vi "室内外单幅图像-阈值设定.vi"() -> ()   [LabVIEW 2018]
uses:
  <vilib>/vision/Image Controls.llb/IMAQ Image.ctl
  <vilib>/Utility/error.llb/DialogType.ctl
  <vilib>/Utility/file.llb/Write Delimited Spreadsheet (I64).vi
  <vilib>/vision/NI_Vision_Development_Module.lvlib
panel:
  out "?":T1(plugin-control)
  in  "刷新按钮":bool
  in  "停止运算":bool
  in  "下一步":bool
  out "Histogram 3":dynamicdata(graph) caption="B直方图"
  out "Histogram 2":dynamicdata(graph) caption="A直方图"
  out "Histogram":dynamicdata(graph) caption="L直方图"
  in  "b颜色通道":cluster{i32, i32}(slide)={-21, 6} scale=-100.0..100.0
  in  "a颜色通道":cluster{i32, i32}(slide)={-21, -7} scale=-100.0..100.0
  in  "L颜色通道":cluster{i32, i32}(slide)={81, 99} scale=0.0..100.0
  out "lie":i32
  out "hang":i32
  out "颜色空间处理后的图，提取火焰":T1(plugin-control)
  in  "Image 4":T1
  out "B":u8[][](array[numeric])
  out "G":u8[][](array[numeric])
  out "R":u8[][](array[numeric])
  out "原图":T1(plugin-control)
  # "Lab颜色空间阈值选择"
  # "Lab颜色分割图像"
  # "滤波平滑图像"
  # "原图"
  # "阈\n值\n选\n择"
  # "火\n焰\n颜\n色\n直\n方\n图"
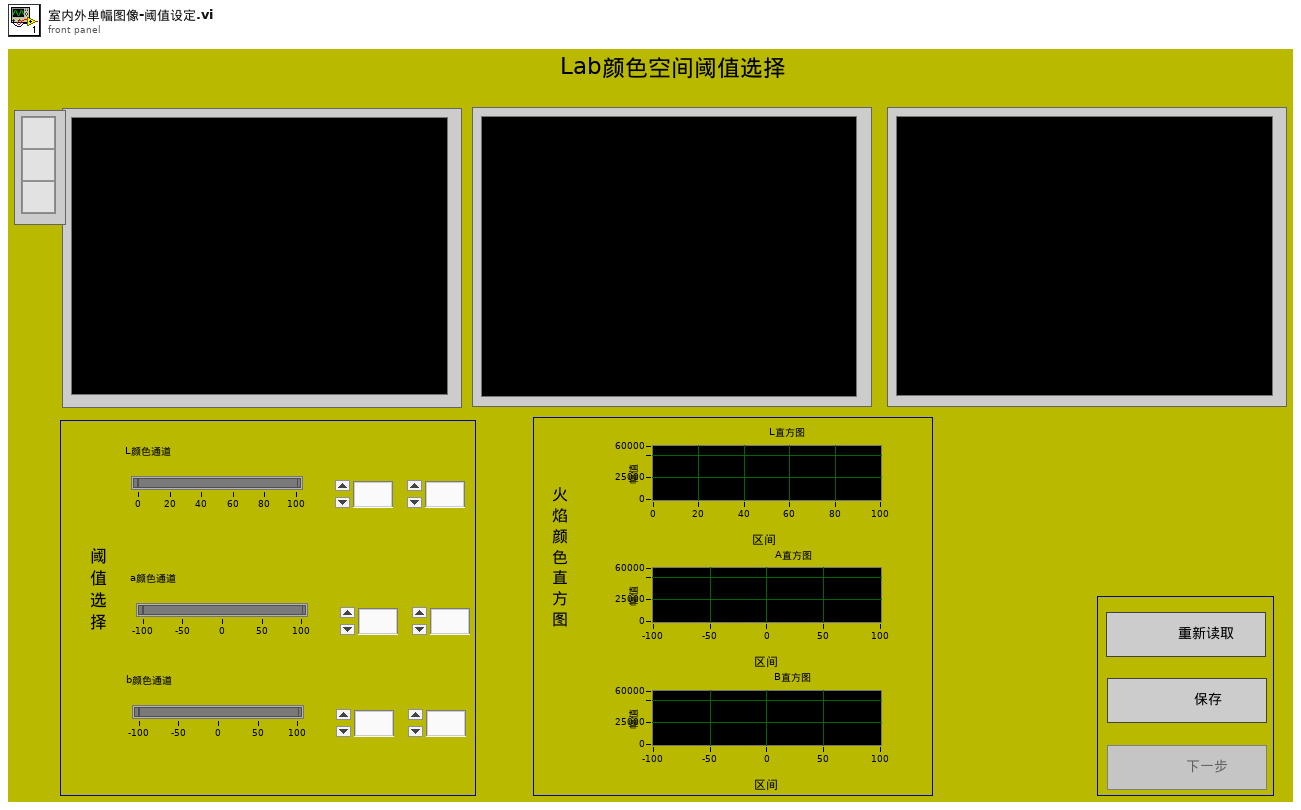
[diagram p1: front panel]
types:
  T1 = typedef "IMAQ Image.ctl" = refnum<image>
  T2 = enum8{"Enabled", "Disabled", "Disabled and Grayed Out"}
  T3 = enum32{"Invalid", "Standard", "Closed", "Hidden", "Minimized", "Maximized"}
  T4 = typedef "Image Type" = u32
  T5 = typedef "DialogType.ctl" = u16
  T6 = cluster{"Global Rectangle":i32[], "Contours":cluster{"Contour Type":u32, "ROI Type":u32, "Points":i32[]}[]}
  T7 = typedef "IMAQ Rectangle" = cluster{"Left":i32, "Top":i32, "Right":i32, "Bottom":i32, "Rotation":dbl}
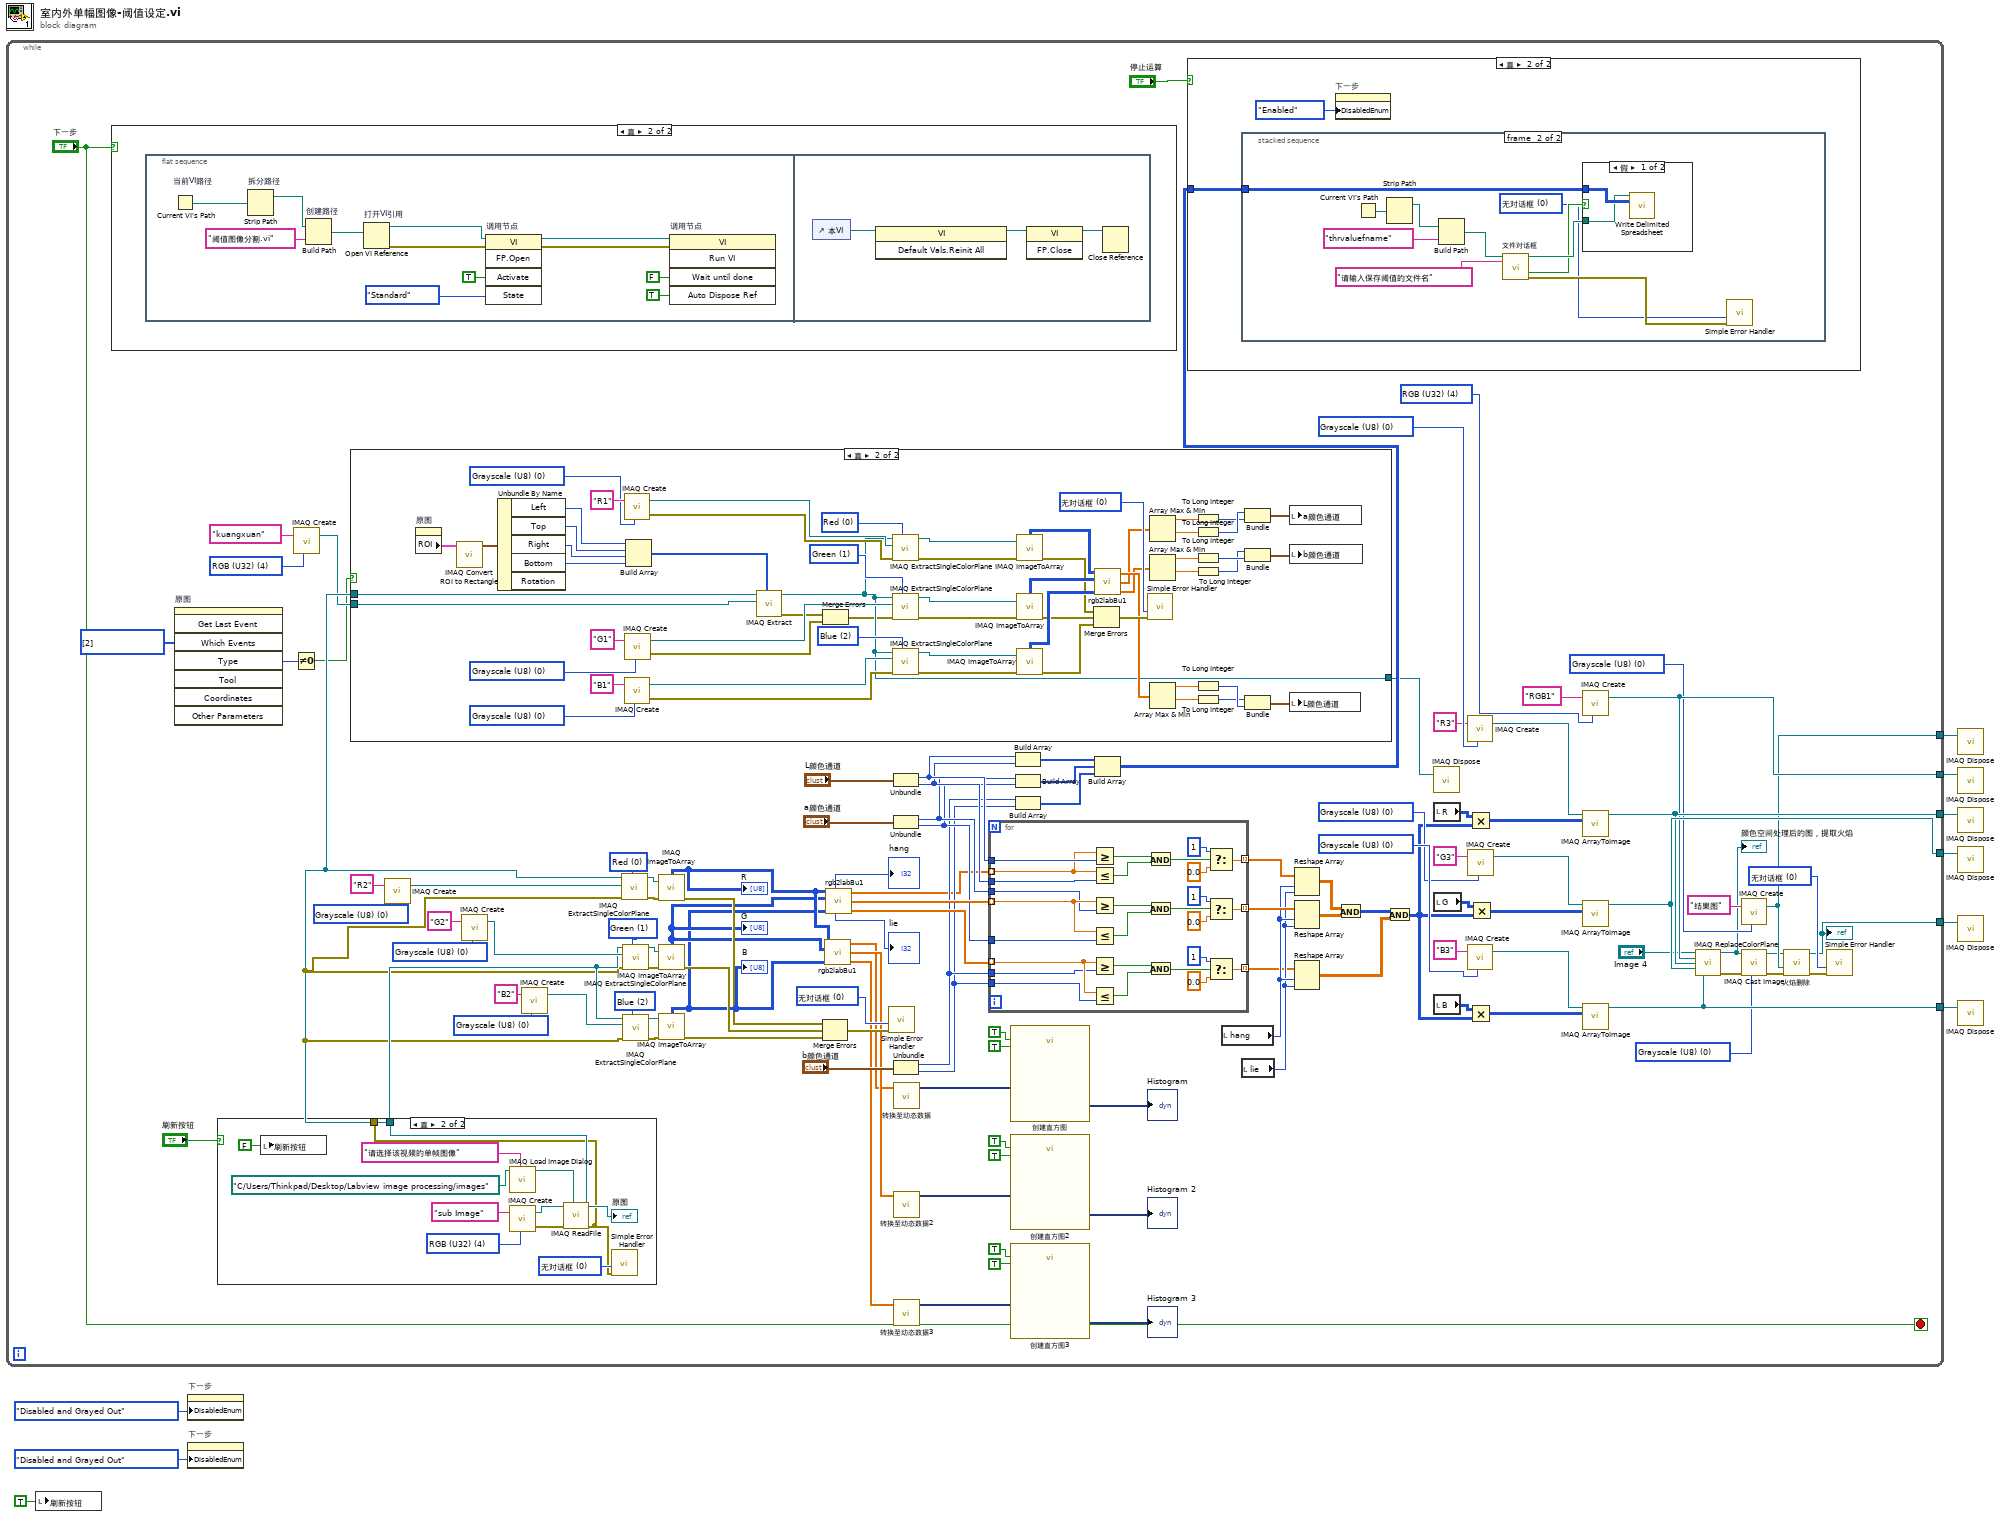
[diagram p0: block diagram]
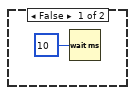
[diagram p2: hidden frame]
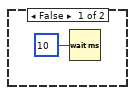
[diagram p3: hidden frame]
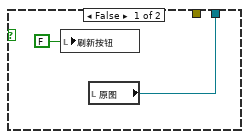
[diagram p4: hidden frame]
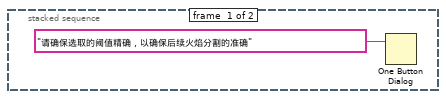
[diagram p6: hidden frame]
diagram:
  n1 = while {
    tunnel: [w123] -> w8
    tunnel: [w122] -> w7
    tunnel: [w121] -> w6
    tunnel: [w120] -> w5
    tunnel: [w119] -> w4
    tunnel: [w11] -> w1
    stop <- "下一步" stop-if-true
    w17 = T4 4 items=["Grayscale (U8)", "Grayscale (I16)", "Grayscale (SGL)", "Complex (CSG)", "RGB (U32)", "HSL (U32)", "RGB (U64)", "Grayscale (U16)"] ("Image Type")
    w16 = i32[] [2] items=["No  event", "Click event", "Draw event", "Move event", "Size event", "Scroll event", "Activate event", "Close event", "Double click event"] ("Events list (all)")
    w28 = T4 0 items=["Grayscale (U8)", "Grayscale (I16)", "Grayscale (SGL)", "Complex (CSG)", "RGB (U32)", "HSL (U32)", "RGB (U64)", "Grayscale (U16)"] ("Image Type")
    w26 = T4 0 items=["Grayscale (U8)", "Grayscale (I16)", "Grayscale (SGL)", "Complex (CSG)", "RGB (U32)", "HSL (U32)", "RGB (U64)", "Grayscale (U16)"] ("Image Type")
    w24 = T4 0 items=["Grayscale (U8)", "Grayscale (I16)", "Grayscale (SGL)", "Complex (CSG)", "RGB (U32)", "HSL (U32)", "RGB (U64)", "Grayscale (U16)"] ("Image Type")
    w54 = T5 0 items=["无对话框", "确定信息", "继续或停止信息", "确定信息＋警告", "继续/停止+警告"] ("type of dialog (OK msg:1)")
    w76 = T4 0 items=["Grayscale (U8)", "Grayscale (I16)", "Grayscale (SGL)", "Complex (CSG)", "RGB (U32)", "HSL (U32)", "RGB (U64)", "Grayscale (U16)"] ("Image Type")
    w77 = T4 4 items=["Grayscale (U8)", "Grayscale (I16)", "Grayscale (SGL)", "Complex (CSG)", "RGB (U32)", "HSL (U32)", "RGB (U64)", "Grayscale (U16)"] ("Image Type")
    w92 = T4 0 items=["Grayscale (U8)", "Grayscale (I16)", "Grayscale (SGL)", "Complex (CSG)", "RGB (U32)", "HSL (U32)", "RGB (U64)", "Grayscale (U16)"] ("Image Type")
    w98 = T4 0 items=["Grayscale (U8)", "Grayscale (I16)", "Grayscale (SGL)", "Complex (CSG)", "RGB (U32)", "HSL (U32)", "RGB (U64)", "Grayscale (U16)"] ("Image Type")
    w96 = T4 0 items=["Grayscale (U8)", "Grayscale (I16)", "Grayscale (SGL)", "Complex (CSG)", "RGB (U32)", "HSL (U32)", "RGB (U64)", "Grayscale (U16)"] ("Image Type")
    w101 = T4 0 items=["Grayscale (U8)", "Grayscale (I16)", "Grayscale (SGL)", "Complex (CSG)", "RGB (U32)", "HSL (U32)", "RGB (U64)", "Grayscale (U16)"] ("Image Type")
    w103 = T5 0 items=["无对话框", "确定信息", "继续或停止信息", "确定信息＋警告", "继续/停止+警告"] ("type of dialog (OK msg:1)")
    w112 = 2 items=["Red", "Green", "Blue", "Hue", "Saturation", "Luminance", "Value", "Intensity"] ("Color Plane")
    w113 = 1 items=["Red", "Green", "Blue", "Hue", "Saturation", "Luminance", "Value", "Intensity"] ("Color Plane")
    w114 = 0 items=["Red", "Green", "Blue", "Hue", "Saturation", "Luminance", "Value", "Intensity"] ("Color Plane")
    n2 = case shown="真" "下一步" {
      frame False {
        n3 = Wait (ms)(milliseconds to wait=u32 10 ("等待时间（毫秒）")) -> ()  [unwired: 1 out]
      }
      frame True {
        n4 = flat-sequence {
          frame #0 {
            n5 = Current VI's Path "当前VI路径"() -> (path=w133:path)
            n6 = Strip Path "拆分路径"(path=w133) -> (stripped path=w136:path)  [unwired: 1 out]
            n7 = Build Path "创建路径"(base path=w136, name or relative path="阈值图像分割.vi" ("名称或相对路径")) -> (appended path=w134:path)
            n8 = Open VI Reference "打开VI引用"(vi path=w134) -> (vi reference=w131:refnum<vi>, error out=w130:errorcluster)  [unwired: 5 in]
            n9 = invoke on="调用节点" class="VI" method="FP.Open"(reference=w131, error in=w130, "Activate"=TRUE ("激活？"), "State"=T3."Standard" ("状态")) -> (reference out=w129:refnum<vi>, error out=w128:errorcluster)  [unwired: 1 in, 3 out]
            n10 = invoke on="调用节点" class="VI" method="Run VI"(reference=w129, error in=w128, "Wait until done"=FALSE ("结束前等待"), "Auto Dispose Ref"=TRUE ("自动销毁引用")) -> ()  [unwired: 1 in, 5 out]
          }
          frame #1 {
            n11 = control-ref of="本VI"() -> (w139:refnum<vi>)
            n12 = invoke class="VI" method="Default Vals.Reinit All"(reference=w139) -> (reference out=w138:refnum<vi>)  [unwired: 2 in, 2 out]
            n13 = invoke class="VI" method="FP.Close"(reference=w138) -> (reference out=w137:refnum<vi>)  [unwired: 2 in, 2 out]
            n14 = Close Reference(reference=w137) -> ()  [unwired: 1 in, 1 out]
          }
        }
      }
    }
    n15 = invoke on="原图" class="ImageControl" method="Get Last Event"("Which Events"=w16) -> ("Type"=w15:i32)  [unwired: 7 in, 7 out]
    n16 = case shown="真" "刷新按钮" {
      tunnel: [_ w203] -> w10
      tunnel: [w201 w204] -> w20
      frame False {
        n17 = local write "刷新按钮"(FALSE ("布尔")) -> ()
        n18 = local read "原图"() -> (w201:T1)
      }
      frame True {
        w208 = T5 0 items=["无对话框", "确定信息", "继续或停止信息", "确定信息＋警告", "继续/停止+警告"] ("type of dialog (OK msg:1)")
        w211 = T4 4 items=["Grayscale (U8)", "Grayscale (I16)", "Grayscale (SGL)", "Complex (CSG)", "RGB (U32)", "HSL (U32)", "RGB (U64)", "Grayscale (U16)"] ("Image Type")
        n19 = local write "刷新按钮"(FALSE ("布尔")) -> ()
        n20 = call "IMAQ Load Image Dialog"("Prompt"="请选择该视频的单帧图像", "Start Path"=path "C:/Users/Thinkpad/Desktop/Labview image processing/images") -> ("Path"=w205:path)  [unwired: 7 in, 2 out]
        n21 = call "IMAQ Create"("Image Name"="sub Image", "Image Type"=w211) -> ("New Image"=w210:T1, "error out"=w209:errorcluster)  [unwired: 2 in, 1 out]
        n22 = call "IMAQ ReadFile"("File Path"=w205, "error in (no error)"=w209, "Image"=w210) -> ("error out"=w203:errorcluster, "Image Out"=w204:T1)  [unwired: 4 in, 3 out]
        "原图" <- w204
        n23 = call <vilib>:"Simple Error Handler.vi"("type of dialog (OK msg:1)"=w208, "error in (no error)"=w203) -> ()  [unwired: 3 in, 5 out]
      }
    }
    n24 = call "IMAQ Create"("Image Name"="kuangxuan", "Image Type"=w17) -> ("New Image"=w19:T1)  [unwired: 2 in, 2 out]
    n25 = Not Equal To 0?(x=w15) -> (x != 0?=w14:bool)
    n26 = case shown="真" w14 {
      tunnel: w19 -> [_ w146]
      tunnel: [_ w145] -> w13
      tunnel: w20 -> [_ w144]
      frame False {
        n27 = Wait (ms)(milliseconds to wait=u32 10) -> ()  [unwired: 1 out]
      }
      frame True {
        w176 = T5 0 items=["无对话框", "确定信息", "继续或停止信息", "确定信息＋警告", "继续/停止+警告"] ("type of dialog (OK msg:1)")
        w187 = 2 items=["Red", "Green", "Blue", "Hue", "Saturation", "Luminance", "Value", "Intensity"] ("Color Plane")
        w188 = 1 items=["Red", "Green", "Blue", "Hue", "Saturation", "Luminance", "Value", "Intensity"] ("Color Plane")
        w189 = 0 items=["Red", "Green", "Blue", "Hue", "Saturation", "Luminance", "Value", "Intensity"] ("Color Plane")
        w193 = T4 0 items=["Grayscale (U8)", "Grayscale (I16)", "Grayscale (SGL)", "Complex (CSG)", "RGB (U32)", "HSL (U32)", "RGB (U64)", "Grayscale (U16)"] ("Image Type")
        w195 = T4 0 items=["Grayscale (U8)", "Grayscale (I16)", "Grayscale (SGL)", "Complex (CSG)", "RGB (U32)", "HSL (U32)", "RGB (U64)", "Grayscale (U16)"] ("Image Type")
        w197 = T4 0 items=["Grayscale (U8)", "Grayscale (I16)", "Grayscale (SGL)", "Complex (CSG)", "RGB (U32)", "HSL (U32)", "RGB (U64)", "Grayscale (U16)"] ("Image Type")
        n28 = property on="原图" class="ImageControl"() -> ("ROI"=w147:T6)  [unwired: 2 in, 2 out]
        n29 = call "IMAQ Convert ROI to Rectangle"("ROI Descriptor"=w147) -> ("Rectangle"=w153:T7)  [unwired: 8 in, 1 out]
        n30 = Unbundle By Name(w153) -> ("Left"=w152:i32, "Top"=w151:i32, "Right"=w150:i32, "Bottom"=w149:i32)  [unwired: 1 out]
        n31 = call "IMAQ Create"("Image Name"="R1", "Image Type"=w197) -> ("New Image"=w192:T1, "error out"=w182:errorcluster)  [unwired: 2 in, 1 out]
        n32 = call "IMAQ Create"("Image Name"="B1", "Image Type"=w193) -> ("New Image"=w190:T1, "error out"=w199:errorcluster)  [unwired: 2 in, 1 out]
        n33 = call "IMAQ Create"("Image Name"="G1", "Image Type"=w195) -> ("New Image"=w191:T1, "error out"=w142:errorcluster)  [unwired: 2 in, 1 out]
        n34 = Build Array(w152, w151, w150, w149) -> (w148:i32[])
        n35 = call "IMAQ Extract"("Optional Rectangle"=w148, "Image Dst"=w146, "Image Src"=w144) -> ("error out"=w143:errorcluster, "Image Dst Out"=w145:T1)  [unwired: 7 in]
        n36 = Merge Errors(w143, w142) -> (w141:errorcluster)
        n37 = call "IMAQ ExtractSingleColorPlane"("Color Plane"=w189, "error in (no error)"=w182, "Image Dst"=w192, "Image Src"=w145) -> ("error out"=w181:errorcluster, "Image Dst Out"=w156:T1)  [unwired: 6 in]
        n38 = call "IMAQ ExtractSingleColorPlane"("Color Plane"=w188, "error in (no error)"=w141, "Image Dst"=w191, "Image Src"=w145) -> ("error out"=w183:errorcluster, "Image Dst Out"=w155:T1)  [unwired: 6 in]
        n39 = call "IMAQ ExtractSingleColorPlane"("Color Plane"=w187, "error in (no error)"=w199, "Image Dst"=w190, "Image Src"=w145) -> ("error out"=w180:errorcluster, "Image Dst Out"=w154:T1)  [unwired: 6 in]
        n40 = call "IMAQ ImageToArray"("error in (no error)"=w181, "Image"=w156) -> ("error out"=w179:errorcluster, "Image Pixels (U8)"=w186:u8[][])  [unwired: 2 in, 3 out]
        n41 = call "IMAQ ImageToArray"("error in (no error)"=w183, "Image"=w155) -> ("error out"=w178:errorcluster, "Image Pixels (U8)"=w185:u8[][])  [unwired: 2 in, 3 out]
        n42 = call "IMAQ ImageToArray"("error in (no error)"=w180, "Image"=w154) -> ("error out"=w177:errorcluster, "Image Pixels (U8)"=w184:u8[][])  [unwired: 2 in, 3 out]
        n43 = Merge Errors(w179, w178, w177) -> (w175:errorcluster)
        n44 = call "rgb2labBu1.vi"("R"=w186, "G"=w185, "B"=w184) -> ("LZ"=w169:dbl[], "aZ"=w158:dbl[], "bZ"=w157:dbl[])  [unwired: 1 in, 2 out]
        n45 = call <vilib>:"Simple Error Handler.vi"("type of dialog (OK msg:1)"=w176, "error in (no error)"=w175) -> ()  [unwired: 3 in, 5 out]
        n46 = Array Max & Min(array=w158) -> (max value=w164:dbl, min value=w165:dbl)  [unwired: 2 out]
        n47 = Array Max & Min(array=w157) -> (max value=w163:dbl, min value=w162:dbl)  [unwired: 2 out]
        n48 = Array Max & Min(array=w169) -> (max value=w174:dbl, min value=w173:dbl)  [unwired: 2 out]
        n49 = To Long Integer(number=w164) -> (32bit integer=w167:i32)
        n50 = To Long Integer(number=w165) -> (32bit integer=w168:i32)
        n51 = To Long Integer(number=w163) -> (32bit integer=w160:i32)
        n52 = To Long Integer(number=w162) -> (32bit integer=w159:i32)
        n53 = To Long Integer(number=w174) -> (32bit integer=w171:i32)
        n54 = To Long Integer(number=w173) -> (32bit integer=w170:i32)
        n55 = Bundle(w168, w167) -> (w166:cluster{i32, i32})  [unwired: 1 in]
        n56 = Bundle(w159, w160) -> (w161:cluster{i32, i32})  [unwired: 1 in]
        n57 = Bundle(w170, w171) -> (w172:cluster{i32, i32})  [unwired: 1 in]
        n58 = local write "a颜色通道"(w166) -> ()
        n59 = local write "b颜色通道"(w161) -> ()
        n60 = local write "L颜色通道"(w172) -> ()
      }
    }
    n61 = call "IMAQ Create"("Image Name"="R2", "Image Type"=w24) -> ("New Image"=w21:T1)  [unwired: 2 in, 2 out]
    n62 = call "IMAQ Create"("Image Name"="G2", "Image Type"=w26) -> ("New Image"=w22:T1)  [unwired: 2 in, 2 out]
    n63 = call "IMAQ Create"("Image Name"="B2", "Image Type"=w28) -> ("New Image"=w23:T1)  [unwired: 2 in, 2 out]
    n64 = call "IMAQ ExtractSingleColorPlane"("Color Plane"=w114, "error in (no error)"=w10, "Image Dst"=w21, "Image Src"=w20) -> ("error out"=w108:errorcluster, "Image Dst Out"=w118:T1)  [unwired: 6 in]
    n65 = call "IMAQ ExtractSingleColorPlane"("Color Plane"=w113, "error in (no error)"=w10, "Image Dst"=w22, "Image Src"=w20) -> ("error out"=w109:errorcluster, "Image Dst Out"=w117:T1)  [unwired: 6 in]
    n66 = call "IMAQ ExtractSingleColorPlane"("Color Plane"=w112, "error in (no error)"=w10, "Image Dst"=w23, "Image Src"=w20) -> ("error out"=w107:errorcluster, "Image Dst Out"=w52:T1)  [unwired: 6 in]
    n67 = call "IMAQ ImageToArray"("error in (no error)"=w108, "Image"=w118) -> ("error out"=w106:errorcluster, "Image Pixels (U8)"=w40:u8[][])  [unwired: 2 in, 3 out]
    "R" <- w40
    n68 = call "IMAQ ImageToArray"("error in (no error)"=w109, "Image"=w117) -> ("error out"=w105:errorcluster, "Image Pixels (U8)"=w39:u8[][])  [unwired: 2 in, 3 out]
    "G" <- w39
    n69 = call "IMAQ ImageToArray"("error in (no error)"=w107, "Image"=w52) -> ("error out"=w104:errorcluster, "Image Pixels (U8)"=w38:u8[][])  [unwired: 2 in, 3 out]
    "B" <- w38
    n70 = Merge Errors(w106, w105, w104) -> (w102:errorcluster)
    n71 = call "rgb2labBu1.vi"("R"=w40, "G"=w39, "B"=w38) -> ("LZ"=w37:dbl[], "aZ"=w42:dbl[], "bZ"=w46:dbl[])  [unwired: 1 in, 2 out]
    n72 = call "rgb2labBu1.vi"("R"=w40, "G"=w39, "B"=w38) -> ("hang"=→"hang":i32, "lie"=→"lie":i32, "LZ"=w51:dbl[], "aZ"=w115:dbl[], "bZ"=w116:dbl[])  [unwired: 1 in]
    n73 = call <vilib>:"Simple Error Handler.vi"("type of dialog (OK msg:1)"=w103, "error in (no error)"=w102) -> ()  [unwired: 3 in, 5 out]
    n74 = Unbundle("L颜色通道") -> (w66:i32, w65:i32)
    n75 = Unbundle("a颜色通道") -> (w64:i32, w63:i32)
    n76 = Unbundle("b颜色通道") -> (w62:i32, w61:i32)
    n77 = call "转换至动态数据"("Array"=w37) -> ("Dynamic Data Type"=w41:dynamicdata)  [unwired: 3 in]
    n78 = call "转换至动态数据2"("Array"=w42) -> ("Dynamic Data Type"=w43:dynamicdata)  [unwired: 3 in]
    n79 = call "转换至动态数据3"("Array"=w46) -> ("Dynamic Data Type"=w47:dynamicdata)  [unwired: 3 in]
    n80 = for {
      tunnel: w51 -> [w247] mode=indexing
      tunnel: w66 -> [w249]
      tunnel: w65 -> [w250]
      tunnel: [w251] -> w74 mode=indexing
      tunnel: w115 -> [w235] mode=indexing
      tunnel: w116 -> [w234] mode=indexing
      tunnel: w64 -> [w233]
      tunnel: w63 -> [w232]
      tunnel: w62 -> [w231]
      tunnel: w61 -> [w230]
      tunnel: [w229] -> w72 mode=indexing
      tunnel: [w228] -> w69 mode=indexing
      n81 = Greater Or Equal?(x=w247, y=w249) -> (x >= y?=w254:bool)
      n82 = Less Or Equal?(x=w247, y=w250) -> (x <= y?=w253:bool)
      n83 = Greater Or Equal?(x=w235, y=w233) -> (x >= y?=w245:bool)
      n84 = Less Or Equal?(x=w235, y=w232) -> (x <= y?=w244:bool)
      n85 = Greater Or Equal?(x=w234, y=w231) -> (x >= y?=w240:bool)
      n86 = Less Or Equal?(x=w234, y=w230) -> (x <= y?=w239:bool)
      n87 = And(x=w254, y=w253) -> (x .and. y?=w252:bool)
      n88 = And(x=w245, y=w244) -> (x .and. y?=w243:bool)
      n89 = And(x=w240, y=w239) -> (x .and. y?=w238:bool)
      n90 = Select(t=1, s=w252, f=0.0) -> (s? t:f=w251:dbl)
      n91 = Select(t=1, s=w243, f=0.0) -> (s? t:f=w229:dbl)
      n92 = Select(t=1, s=w238, f=0.0) -> (s? t:f=w228:dbl)
    }
    n93 = call "创建直方图"("Reset"=TRUE, "Enable"=TRUE, "Signal"=w41) -> ("Histogram"=→"Histogram":dynamicdata)  [unwired: 7 in, 1 out]
    n94 = call "创建直方图2"("Reset"=TRUE, "Enable"=TRUE, "Signal"=w43) -> ("Histogram"=→"Histogram 2":dynamicdata)  [unwired: 7 in, 1 out]
    n95 = call "创建直方图3"("Reset"=TRUE, "Enable"=TRUE, "Signal"=w47) -> ("Histogram"=→"Histogram 3":dynamicdata)  [unwired: 7 in, 1 out]
    n96 = Build Array(w66, w65) -> (w60:i32[])
    n97 = Build Array(w64, w63) -> (w59:i32[])
    n98 = Build Array(w62, w61) -> (w58:i32[])
    n99 = Build Array(w60, w59, w58) -> (w57:i32[][])
    n100 = case shown="真" "停止运算" {
      tunnel: w57 -> [_ w214]
      frame False {
      }
      frame True {
        n101 = stacked-sequence {
          tunnel: w214 -> [_ w225]
          frame #0 {
            n102 = One Button Dialog(message="请确保选取的阈值精确，以确保后续火焰分割的准确" ("消息")) -> ()  [unwired: 1 in, 1 out]
          }
          frame #1 {
            w217 = T5 0 items=["无对话框", "确定信息", "继续或停止信息", "确定信息＋警告", "继续/停止+警告"] ("type of dialog (OK msg:1)")
            n103 = Current VI's Path() -> (path=w222:path)
            n104 = Strip Path(path=w222) -> (stripped path=w223:path)  [unwired: 1 out]
            n105 = Build Path(base path=w223, name or relative path="thrvaluefname" ("名称或相对路径")) -> (appended path=w221:path)
            n106 = call "文件对话框"("start path"=w221, "prompt"="请输入保存阈值的文件名") -> ("selected path"=w220:path, "cancelled"=w219:bool, "error out"=w218:errorcluster)  [unwired: 10 in, 1 out]
            n107 = case shown="假" w219 {
              tunnel: w225 -> [w227 _]
              tunnel: w220 -> [w226 _]
              frame False {
                n108 = call-poly <vilib>:"Write Delimited Spreadsheet.vi"("file path (dialog if empty)"=w226, "2D data"=w227) -> ()  [unwired: 12 in, 2 out]
              }
              frame True {
              }
            }
            n109 = call <vilib>:"Simple Error Handler.vi"("type of dialog (OK msg:1)"=w217, "error in (no error)"=w218) -> ()  [unwired: 3 in, 5 out]
          }
        }
        n110 = property on="下一步" class="Bool"("DisabledEnum"=T2."Enabled" ("禁用")) -> ()  [unwired: 2 in, 2 out]
      }
    }
    n111 = local read "hang"() -> (w71:i32)
    n112 = local read "lie"() -> (w70:i32)
    n113 = Reshape Array(w74, w71, w70) -> (w73:dbl[][])
    n114 = Reshape Array(w72, w71, w70) -> (w67:dbl[][])
    n115 = Reshape Array(w69, w71, w70) -> (w68:dbl[][])
    n116 = And(x=w73, y=w67) -> (x .and. y?=w90:i32[][])
    n117 = And(x=w90, y=w68) -> (x .and. y?=w83:i32[][])
    n118 = call "IMAQ Dispose"("Image"=w13) -> ()  [unwired: 5 in, 1 out]
    n119 = local read "R"() -> (w89:u8[][])
    n120 = local read "G"() -> (w88:u8[][])
    n121 = local read "B"() -> (w87:u8[][])
    n122 = call "IMAQ Create"("Image Name"="R3", "Image Type"=w101) -> ("New Image"=w99:T1)  [unwired: 2 in, 2 out]
    n123 = call "IMAQ Create"("Image Name"="B3", "Image Type"=w98) -> ("New Image"=w93:T1)  [unwired: 2 in, 2 out]
    n124 = Multiply(x=w89, y=w83) -> (x*y=w86:i32[][])
    n125 = call "IMAQ Create"("Image Name"="G3", "Image Type"=w96) -> ("New Image"=w94:T1)  [unwired: 2 in, 2 out]
    n126 = Multiply(x=w87, y=w83) -> (x*y=w84:i32[][])
    n127 = Multiply(x=w88, y=w83) -> (x*y=w85:i32[][])
    n128 = call "IMAQ Create"("Image Name"="RGB1", "Image Type"=w77) -> ("New Image"=w120:T1)  [unwired: 2 in, 2 out]
    n129 = call "IMAQ ArrayToImage"("Image Pixels (U8)"=w86, "Image"=w99) -> ("Image Out"=w121:T1)  [unwired: 8 in, 1 out]
    n130 = call "IMAQ ArrayToImage"("Image Pixels (U8)"=w85, "Image"=w94) -> ("Image Out"=w122:T1)  [unwired: 8 in, 1 out]
    n131 = call "IMAQ ArrayToImage"("Image Pixels (U8)"=w84, "Image"=w93) -> ("Image Out"=w123:T1)  [unwired: 8 in, 1 out]
    n132 = call "IMAQ ReplaceColorPlane"("Image Src"="Image 4", "Image Dst"=w120, "Red or Hue Plane"=w121, "Green or Sat Plane"=w122, "Blue or Luma or Val or Inten Plane"=w123) -> ("Image Dst Out"=w75:T1, "error out"=w56:errorcluster)  [unwired: 9 in]
    "颜色空间处理后的图，提取火焰" <- w75
    n133 = call "IMAQ Create"("Image Name"="结果图", "Image Type"=w92) -> ("New Image"=w119:T1)  [unwired: 2 in, 2 out]
    n134 = call "IMAQ Cast Image"("Image Type"=w76, "error in (no error)"=w56, "Image Src"=w75) -> ("error out"=w55:errorcluster, "Image Dst Out"=w79:T1)  [unwired: 7 in]
    n135 = call "火焰删除.vi"("error in (no error)"=w55, "Image dst"=w119, "Image source"=w79) -> ("error out"=w53:errorcluster, "Threshold Image"=w11:T1)  [unwired: 7 in]
    "?" <- w11
    n136 = call <vilib>:"Simple Error Handler.vi"("type of dialog (OK msg:1)"=w54, "error in (no error)"=w53) -> ()  [unwired: 3 in, 5 out]
  }
  n137 = local write "刷新按钮"(TRUE ("布尔")) -> ()
  n138 = property on="下一步" class="Bool"("DisabledEnum"=T2."Disabled and Grayed Out" ("禁用")) -> ()  [unwired: 2 in, 2 out]
  n139 = property on="下一步" class="Bool"("DisabledEnum"=T2."Disabled and Grayed Out" ("禁用")) -> ()  [unwired: 2 in, 2 out]
  n140 = call "IMAQ Dispose"("Image"=w4) -> ()  [unwired: 5 in, 1 out]
  n141 = call "IMAQ Dispose"("Image"=w5) -> ()  [unwired: 5 in, 1 out]
  n142 = call "IMAQ Dispose"("Image"=w6) -> ()  [unwired: 5 in, 1 out]
  n143 = call "IMAQ Dispose"("Image"=w7) -> ()  [unwired: 5 in, 1 out]
  n144 = call "IMAQ Dispose"("Image"=w1) -> ()  [unwired: 5 in, 1 out]
  n145 = call "IMAQ Dispose"("Image"=w8) -> ()  [unwired: 5 in, 1 out]
